vi "Items.vi"(8 "error in (no error)":errorcluster, 11 "ListImp in":refnum<class "ListImp.lvclass">) -> (0 "error out":errorcluster, 1 "Items":refnum<class>[](array[class]), 3 "ListImp out":refnum<class "ListImp.lvclass">)   [LabVIEW 2013, in "LapDog.Collections.v_.Lists.lvlib" / "ListImp.lvclass"]
doc: "Returns a copy of all items in the list."
uses:
  ListImp.lvclass
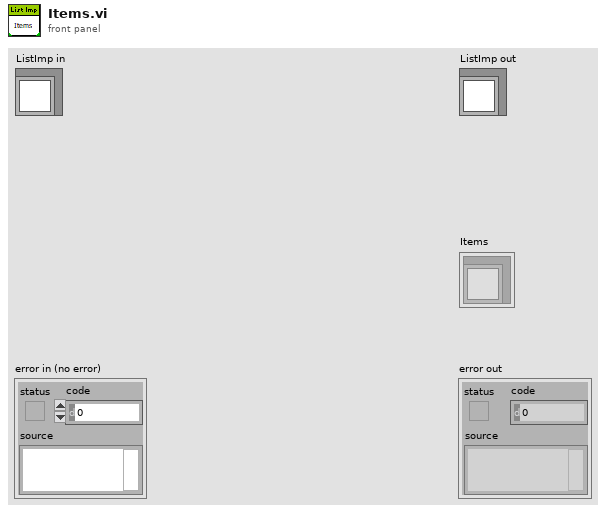
[diagram p1: front panel]
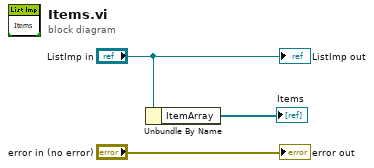
[diagram p0: block diagram]
diagram:
  n1 = Unbundle By Name("ListImp in") -> ("ItemArray"=→"Items":refnum<class>[])
  "error out" <- "error in (no error)"
  "ListImp out" <- "ListImp in"
